vi "Subpanel - Test.vi"() -> ()   [LabVIEW 2016]
uses:
  main/apis/Setup/GetVI/GetVIByPath.vi
  main/apis/Stimulus/VI/OpenVIFrontPanel.vi
  main/apis/Stimulus/VI/RunVI.vi
  main/apis/Stimulus/VI/MakeVIFrontMost.vi
  main/apis/Stimulus/ValueSignal/ValueSignalByPathString.vi
  main/apis/Stimulus/KeyBoardSimulation/ValueSignalLatchBooleanString.vi
  main/Drona.lvlib
  main/apis/Setup/GetVI/GetVI.lvlib
  <vilib>/addons/_JKI Toolkits/Caraya/classes/Test/Test.lvclass
  main/apis/Stimulus/ValueSignal/ValueSignal.lvlib
  main/apis/Stimulus/VI/VI.lvlib
  main/apis/Stimulus/KeyBoardSimulation/KeyboardSimulation.lvlib
panel:
  out "error out":errorcluster
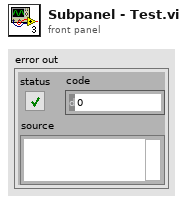
[diagram p1: front panel]
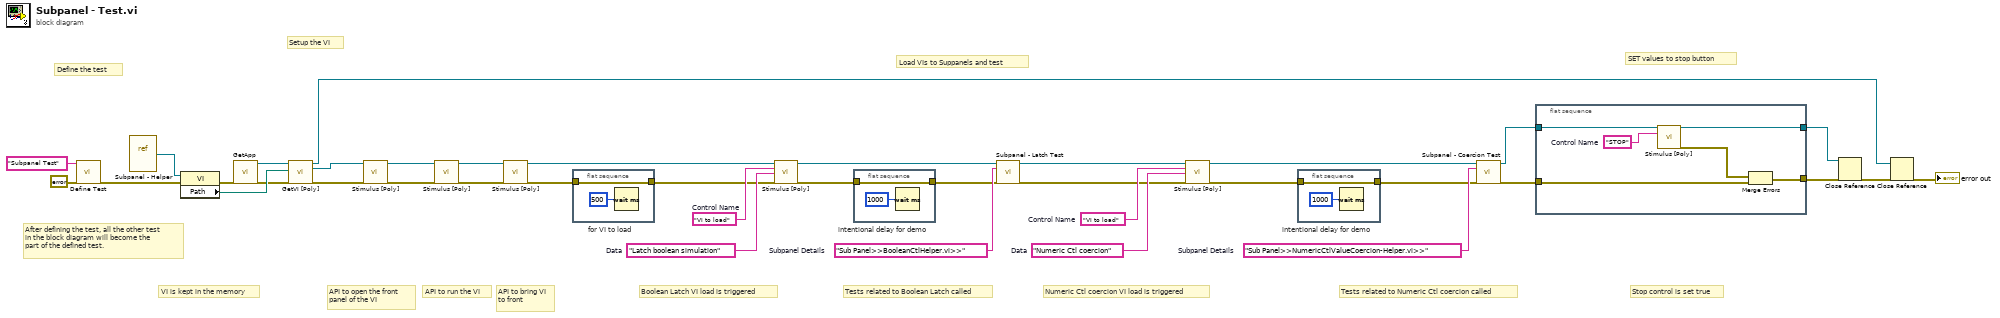
[diagram p0: block diagram]
diagram:
  w14 = "Sub Panel>>BooleanCtlHelper.vi>>"  # Subpanel Details
  w17 = "Latch boolean simulation"  # Data
  w16 = "VI to load"  # Control Name
  w18 = "Sub Panel>>NumericCtlValueCoercion-Helper.vi>>"  # Subpanel Details
  w20 = "Numeric Ctl coercion"  # Data
  w21 = "VI to load"  # Control Name
  # "Load VIs to Suppanels and test"
  # "API to bring VI to front"
  # "Boolean Latch VI load is triggered"
  # "Tests related to Boolean Latch called"
  # "Tests related to Numeric Ctl coercion called"
  # "Numeric Ctl coercion VI load is triggered"
  # "API to open the front\npanel of the VI"
  # "Stop control is set true"
  # "SET values to stop button"
  # "API to run the VI"
  # "VI is kept in the memory"
  # "Setup the VI"
  # "After defining the test, all the other test\nin the block diagram will become the \npart of the defined test."
  # "Define the test"
  n1 = call <vilib>:"Define Test.vi"("error in (no error)"=errorcluster {"status"=FALSE, "code"=0, "source"=""}, "Label (VI Title)"="Subpanel Test") -> ("error out"=w33:errorcluster)  [unwired: 9 in]
  n2 = vi-ref "Subpanel - Helper.vi"() -> (w22:refnum<vi>)
  n3 = property on="Property Node" class="VI"(reference=w22, error in=w33) -> (error out=w37:errorcluster, "Path"=w36:path)  [unwired: 1 out]
  n4 = call "GetApp.vi"("error in (no error)"=w37) -> ("Application Ref"=w38:refnum<vi>, "error out"=w35:errorcluster)  [unwired: 13 in]
  n5 = call-poly "GetVI [Poly].vi"("Application Ref in"=w38, "VI Path"=w36, "error in (no error)"=w35) -> ("Application Ref out"=w23:refnum<vi>, "VI Reference"=w28:refnum<vi>, "error out"=w30:errorcluster)  [unwired: 10 in]
  n6 = call-poly "Stimulus [Poly].vi"("VI Reference In"=w28, "error in"=w30) -> ("VI Reference Out"=w27:refnum<vi>, "error out"=w29:errorcluster)  [unwired: 12 in]
  n7 = call-poly "Stimulus [Poly].vi"("VI Reference In"=w27, "error in"=w29) -> ("VI Reference Out"=w9:refnum<vi>, "error out"=w8:errorcluster)  [unwired: 12 in]
  n8 = call-poly "Stimulus [Poly].vi"("VI Reference In"=w9, "error in"=w8) -> ("VI Reference Out"=w7:refnum<vi>, "error out"=w2:errorcluster)  [unwired: 12 in]
  n9 = flat-sequence "for VI to load" {
    tunnel: w2 -> [w39]
    tunnel: [w39] -> w1
    frame #0 {
      n10 = Wait (ms)(milliseconds to wait=u32 500) -> ()  [unwired: 1 out]
    }
  }
  n11 = call-poly "Stimulus [Poly].vi"("VI Reference In"=w7, "Control Path"=w16, "Value (Signaling)"=w17, "error in"=w1) -> ("VI Reference Out"=w15:refnum<vi>, "error out"=w6:errorcluster)  [unwired: 10 in]
  n12 = flat-sequence "intentional delay for demo" {
    tunnel: w6 -> [w41]
    tunnel: [w41] -> w5
    frame #0 {
      n13 = Wait (ms)(milliseconds to wait=u32 1000) -> ()  [unwired: 1 out]
    }
  }
  n14 = call "Subpanel - Latch Test.vi"("VI Reference In"=w15, "Subpanel Details"=w14, "error in (no error)"=w5) -> ("VI Reference Out"=w13:refnum<vi>, "error out"=w12:errorcluster)  [unwired: 11 in]
  n15 = call-poly "Stimulus [Poly].vi"("VI Reference In"=w13, "Control Path"=w21, "Value (Signaling)"=w20, "error in"=w12) -> ("VI Reference Out"=w19:refnum<vi>, "error out"=w4:errorcluster)  [unwired: 10 in]
  n16 = flat-sequence "intentional delay for demo" {
    tunnel: w4 -> [w43]
    tunnel: [w43] -> w3
    frame #0 {
      n17 = Wait (ms)(milliseconds to wait=u32 1000) -> ()  [unwired: 1 out]
    }
  }
  n18 = call "Subpanel - Coercion Test.vi"("VI Reference In"=w19, "Subpanel Details"=w18, "error in (no error)"=w3) -> ("VI Reference Out"=w10:refnum<vi>, "error out"=w11:errorcluster)  [unwired: 11 in]
  n19 = flat-sequence {
    tunnel: [w49] -> w26
    tunnel: [w50] -> w25
    tunnel: w11 -> [w46]
    tunnel: w10 -> [w45]
    frame #0 {
      w47 = "STOP"  # Control Name
      n20 = call-poly "Stimulus [Poly].vi"("VI Reference In"=w45, "Control Path"=w47) -> ("VI Reference Out"=w50:refnum<vi>, "error out"=w48:errorcluster)  [unwired: 12 in]
      n21 = Merge Errors(w48, w46) -> (w49:errorcluster)
    }
  }
  n22 = Close Reference(reference=w25, error in (no error)=w26) -> (error out=w31:errorcluster)
  n23 = Close Reference(reference=w23, error in (no error)=w31) -> (error out=→"error out":errorcluster)
